vi "thermo_concentrate_results.vi"(1 "array in":dbl[][](array[numeric])) -> (0 "vector out":dbl[](array[numeric]))   [LabVIEW 2020]
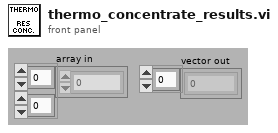
[diagram p1: front panel]
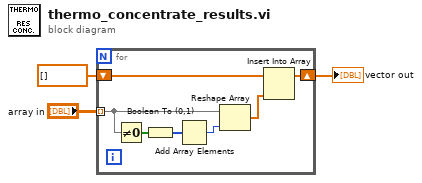
[diagram p0: block diagram]
diagram:
  n1 = for {
    tunnel: "array in" -> [w8] mode=indexing
    shift-right: [w4] -> w1
    shift-left: dbl[] [] -> [w5]
    n2 = Not Equal To 0?(x=w8) -> (x != 0?=w10:bool[])
    n3 = Boolean To (0,1)(Boolean=w10) -> (0, 1=w9:i16[])
    n4 = Add Array Elements(numeric array=w9) -> (sum=w7:i16)
    n5 = Reshape Array(w8, w7) -> (w6:dbl[])
    n6 = Insert Into Array(array=w5, new element=w6) -> (w4:dbl[])  [unwired: 1 in]
  }
  "vector out" <- w1
